vi "findPHSerror——test.vi"() -> ()   [LabVIEW 2016]
uses:
  <vilib>/Utility/file.llb/Write Delimited Spreadsheet (DBL).vi
panel:
  in  "osc in":refnum<visa-resource-name>
  out "Real":dbl
  in  "freq (MHz)":dbl=1.367
  in  "HIFU port":u32=12321
  in  "HIFU ip":string="192.168.1.24"
  out "Waveform Graph":dbl[](graph)
  out "channel":dbl
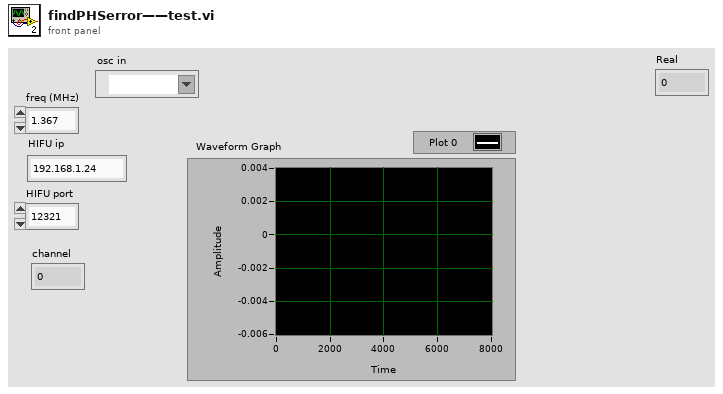
[diagram p1: front panel]
types:
  T1 = typedef "NI_Matrix.lvlib/RealMatrix.ctl" = dbl[][]
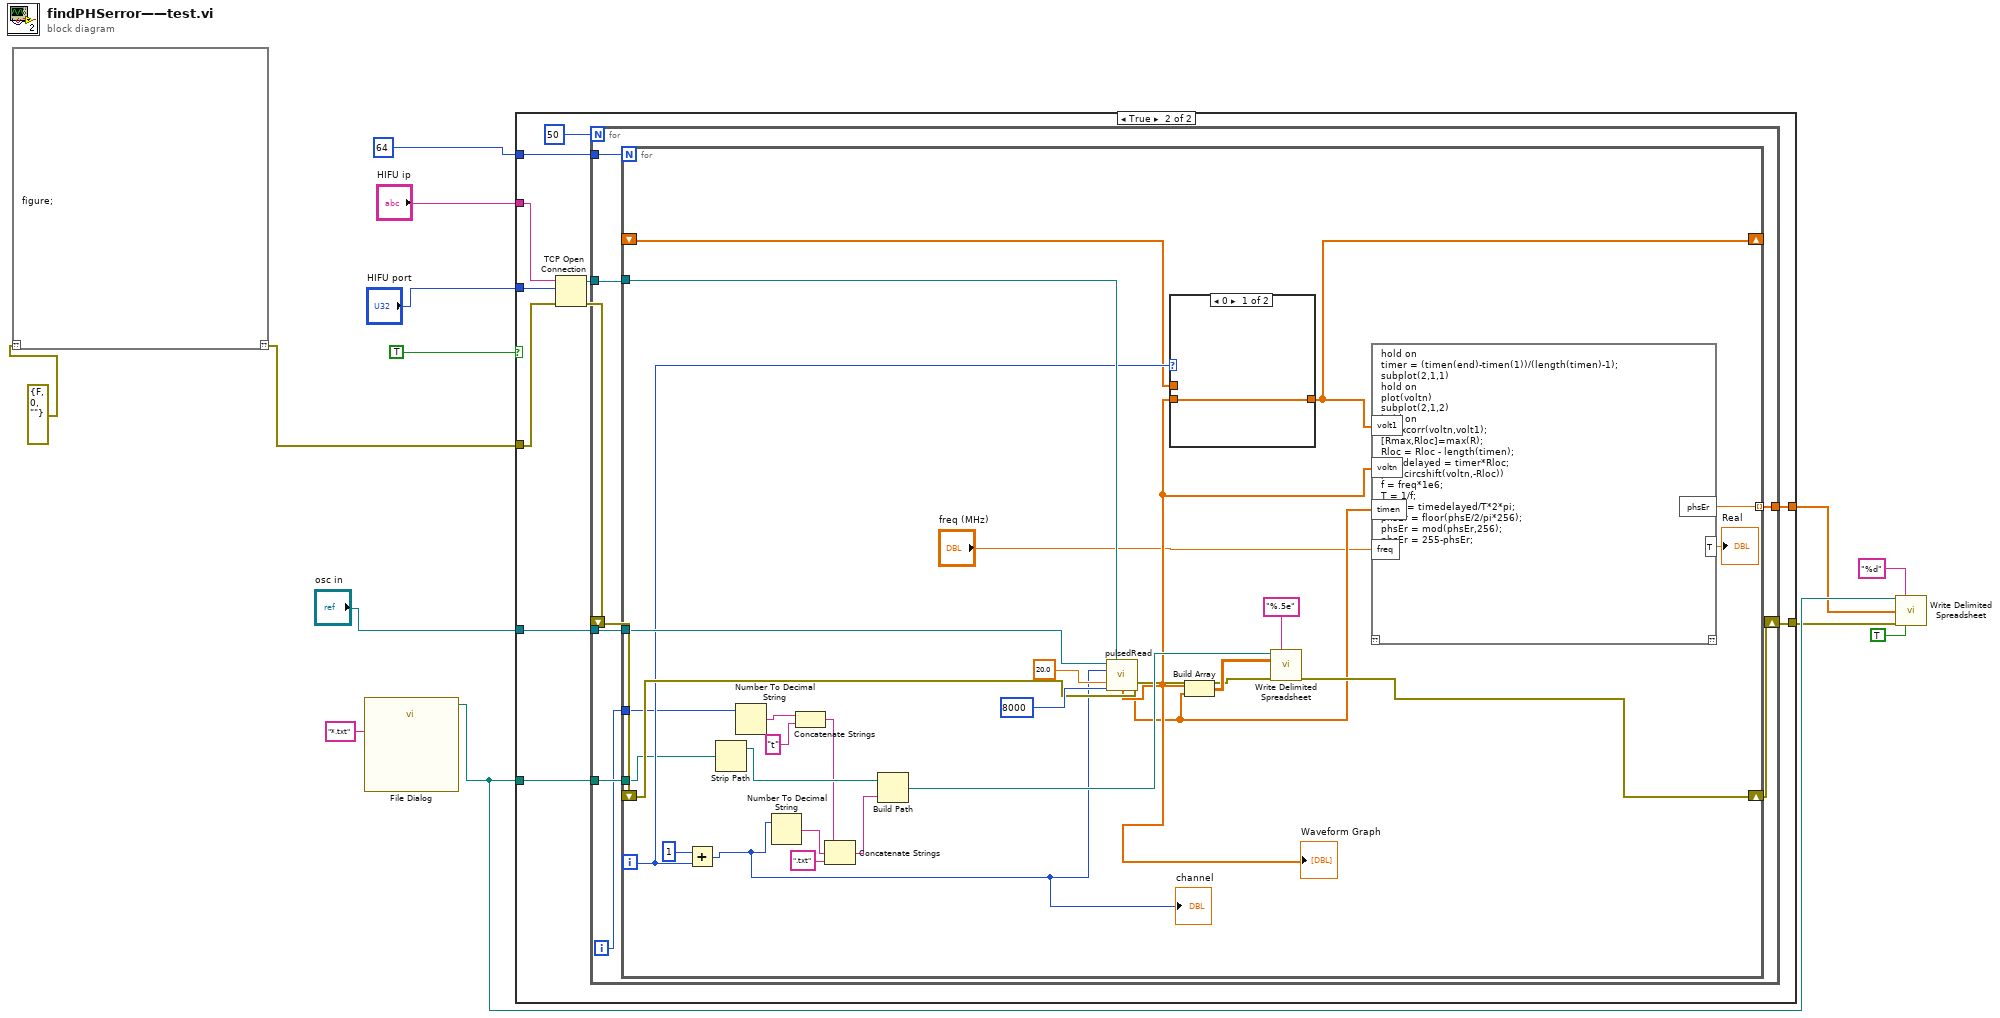
[diagram p0: block diagram]
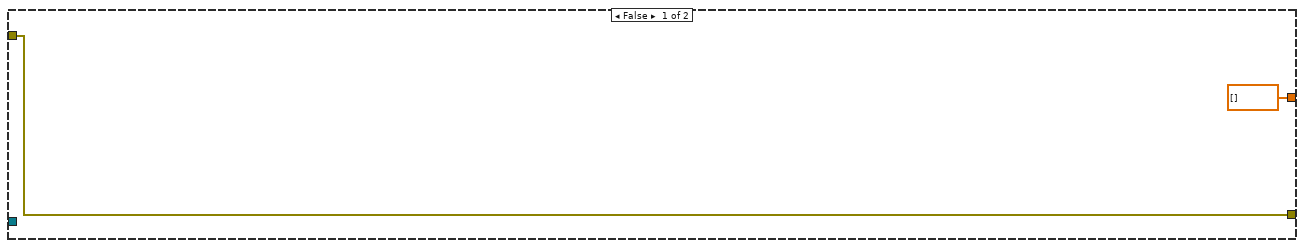
[diagram p2: hidden frame]
diagram:
  n1 = script code="figure;"("??"=errorcluster {"status"=FALSE, "code"=0, "source"=""} ("error out")) -> ("??"=w1:errorcluster)
  n2 = call "File Dialog"("pattern (all files)"="*.txt") -> ("selected path"=w7:path)  [unwired: 11 in, 3 out]
  n3 = case shown="True" TRUE {
    tunnel: 64 -> [_ w26]
    tunnel: w1 -> [w14 w21]
    tunnel: "osc in" -> [_ w25]
    tunnel: w7 -> [_ w24]
    tunnel: "HIFU ip" -> [_ w23]
    tunnel: "HIFU port" -> [_ w22]
    tunnel: [dbl[] [] w18] -> w6
    tunnel: [w14 w17] -> w5
    frame False {
    }
    frame True {
      n4 = TCP Open Connection(address=w23, remote port or service name=w22, error in (no error)=w21) -> (connection ID=w19:refnum<k5>, error out=w20:errorcluster)  [unwired: 2 in]
      n5 = for {
        N: 50 -> [_]
        tunnel: w26 -> [w34]
        tunnel: w25 -> [w33]
        tunnel: w24 -> [w32]
        tunnel: w19 -> [w30]
        tunnel: [w29] -> w18
        shift-right: [w28] -> w17
        shift-left: w20 -> [w31]
        i -> [w27]
        n6 = for {
          N: w34 -> [_]
          tunnel: w33 -> [w53]
          tunnel: w32 -> [w41]
          shift-right: [w52] -> w28
          shift-left: w31 -> [w54]
          tunnel: w30 -> [w50]
          shift-right: [w46] -> _
          shift-left: _ -> [w47]
          tunnel: [w42] -> w29 mode=indexing
          tunnel: w27 -> [w38]
          i -> [w48]
          n7 = Add(x=1, y=w48) -> (x+y=w49:i32)
          "channel" <- w49
          n8 = Strip Path(path=w41) -> (stripped path=w40:path)  [unwired: 1 out]
          n9 = Number To Decimal String(number=w38) -> (decimal integer string=w37:string)  [unwired: 1 in]
          n10 = Number To Decimal String(number=w49) -> (decimal integer string=w59:string)  [unwired: 1 in]
          n11 = Concatenate Strings(w37, "t" ("string")) -> (w35:string)
          n12 = Concatenate Strings(w35, w59, ".txt" ("string")) -> (w58:string)
          n13 = Build Path(base path=w40, name or relative path=w58) -> (appended path=w57:path)
          n14 = call "pulsedRead.vi"("osc in"=w53, "connection ID"=w50, "channel"=w49, "error in (no error)"=w54, "cycles"=20.0, "points"=u64 8000) -> ("error out"=w55:errorcluster, "voltage"=w45:dbl[], "time"=w44:dbl[])  [unwired: 4 in, 3 out]
          "Waveform Graph" <- w45
          n15 = case shown="0" w48 {
            tunnel: w45 -> [w64 _]
            tunnel: [w64 w65] -> w46
            tunnel: w47 -> [_ w65]
            frame 0 {
            }
            frame 1, Default {
            }
          }
          n16 = Build Array(w45, w44) -> (w56:T1)
          n17 = call-poly <vilib>:"Write Delimited Spreadsheet.vi"("file path (dialog if empty)"=w57, "format (%.3f)"="%.5e", "2D data"=w56, "error in (no error)"=w55) -> ("error out"=w52:errorcluster)  [unwired: 10 in, 1 out]
          n18 = script code="hold on\ntimer = (timen(end)-timen(1))/(length(timen)-1);\nsubplot(2,1,1)\nhold on\nplot(voltn)\nsubplot(2,1,2)\nhold on\nR = xcorr(voltn,volt1);\n[Rmax,Rloc]=max(R);\nRloc = Rloc - length(timen);\ntimedelayed = timer*Rloc;\nplot(circshift(voltn,-Rloc))\nf = freq*1e6;\nT = 1/f;\nphsE = timedelayed/T*2*pi;\nphsEr = floor(phsE/2/pi*256);\nphsEr = mod(phsEr,256);\nphsEr = 255-phsEr;"("volt1"=w46, "voltn"=w45, "timen"=w44, "freq"="freq (MHz)") -> ("phsEr"=w42:dbl, "T"=→"Real":dbl)  [unwired: 1 in, 1 out]
        }
      }
    }
  }
  n19 = call-poly <vilib>:"Write Delimited Spreadsheet.vi"("file path (dialog if empty)"=w7, "format (%.3f)"="%d", "1D data"=w6, "error in (no error)"=w5, "transpose? (no:F)"=TRUE) -> ()  [unwired: 9 in, 2 out]
